vi "mymodule2.vi"() -> ()   [LabVIEW 2018]
uses:
  <vilib>/Enthought/Python Integration Toolkit/api/Unpack Double Array.vi
  <vilib>/Enthought/Python Integration Toolkit/Python Integration Toolkit.lvlib
panel:
  in  "停止":bool
  out "Data Out":dbl[](array[numeric])
  in  "OFFSET":dbl
  in  "Call Python":bool
  in  "Scale":dbl
  in  "Data In":dbl[](array[numeric])
  # "Python Global Varables"
  # "Data Out = Data In * Scale + OFFSET"
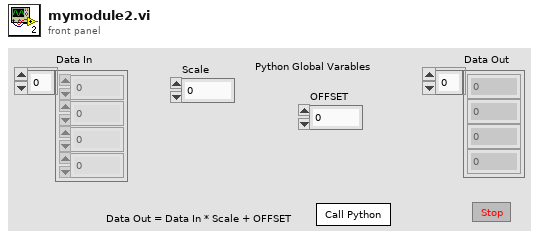
[diagram p1: front panel]
types:
  T1 = typedef "Python Integration Toolkit.lvlib/Session ID.ctl" = u64
  T2 = typedef "Python Integration Toolkit.lvlib/Python Objects.ctl" = variant
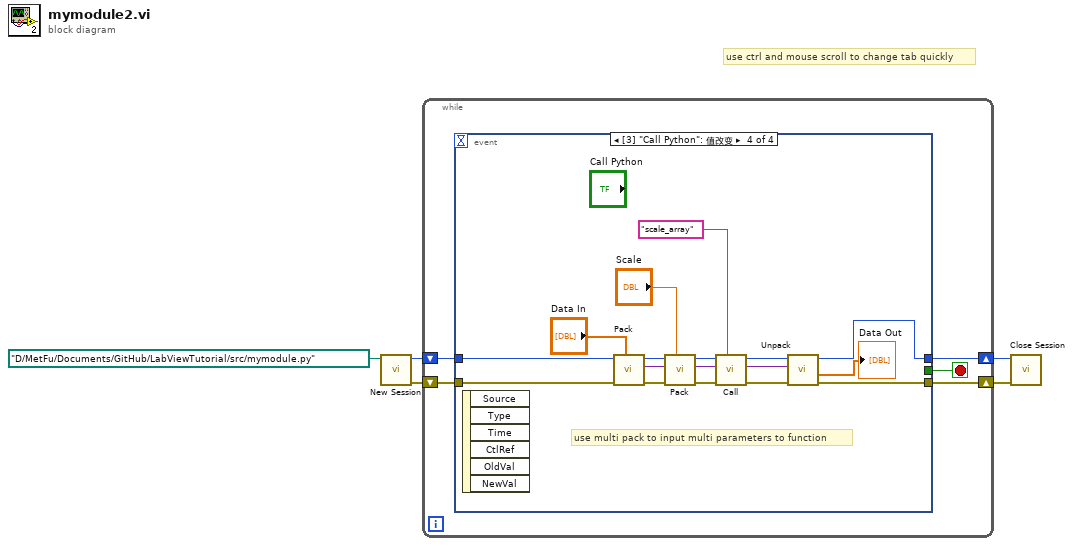
[diagram p0: block diagram]
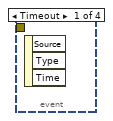
[diagram p2: hidden frame]
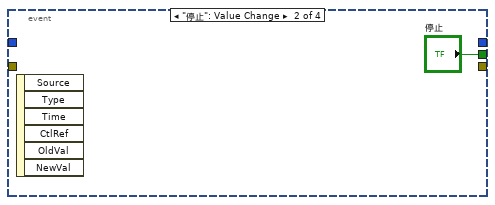
[diagram p3: hidden frame]
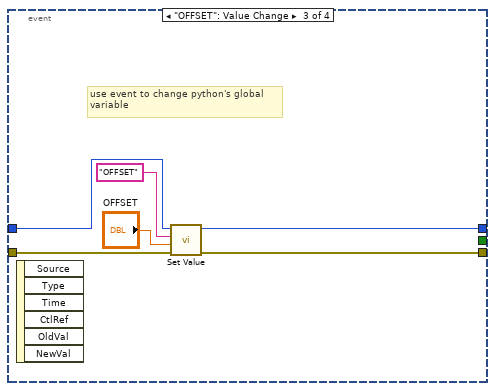
[diagram p4: hidden frame]
diagram:
  # "use ctrl and mouse scroll to change tab quickly"
  n1 = call <vilib>:"New Session.vi"("Path to Python Module (.py File)"=path "D:/MetFu/Documents/GitHub/LabViewTutorial/src/mymodule.py") -> ("error out"=w1:errorcluster, "Session ID out"=w4:T1)  [unwired: 9 in]
  n2 = while {
    shift-right: [w9] -> w3
    shift-left: w4 -> [w10]
    shift-right: [w8] -> w2
    shift-left: w1 -> [w7]
    stop <- w6 stop-if-true
    n3 = event shown="[3] \"Call Python\": 值改变" {
      selector: _ -> [_ _ _ _]
      dyn-events: _ -> [_ _ _ _]
      timeout: _ -> [_ _ _ _]
      tunnel: w10 -> [_ _ w15 w30]
      tunnel: [_ _ w14 w29] -> w9
      tunnel: [_ _ w13 w27] -> w8
      tunnel: w7 -> [_ _ w12 w28]
      tunnel: [_ "停止" _ _] -> w6
      event Timeout {
        n4 = event-data() -> ()  [unwired: 1 in, 3 out]
      }
      event "停止": Value Change {
        n5 = event-data() -> ()  [unwired: 1 in, 6 out]
      }
      event "OFFSET": Value Change {
        # "use event to change python's global\nvariable"
        n6 = event-data() -> ()  [unwired: 1 in, 6 out]
        n7 = call <vilib>:"Set Value.vi"("error in (no error)"=w12, "Value"="OFFSET", "Object Name"="OFFSET", "Session ID"=w15) -> ("error out"=w13:errorcluster, "Session ID out"=w14:T1)  [unwired: 6 in]
      }
      event "Call Python": Value Change {
        # "use multi pack to input multi parameters to function"
        n8 = event-data() -> ()  [unwired: 1 in, 6 out]
        n9 = call <vilib>:"Pack.vi"("Argument"="Data In", "error in (no error)"=w28, "Session ID"=w30) -> ("error out"=w20:errorcluster, "Python Object References Out"=w23:T2, "Session ID out"=w25:T1)  [unwired: 6 in]
        n10 = call <vilib>:"Pack.vi"("Argument"="Scale", "error in (no error)"=w20, "Python Object References In"=w23, "Session ID"=w25) -> ("error out"=w21:errorcluster, "Python Object References Out"=w22:T2, "Session ID out"=w24:T1)  [unwired: 5 in]
        n11 = call <vilib>:"Call.vi"("Function or Method Name"="scale_array", "error in (no error)"=w21, "Python Object References In"=w22, "Session ID"=w24) -> ("error out"=w33:errorcluster, "Python Object References Out"=w34:T2, "Session ID out"=w32:T1)  [unwired: 5 in]
        n12 = call-poly <vilib>:"Unpack.vi"("error in (no error)"=w33, "Python Object References In"=w34, "Session ID"=w32) -> ("error out"=w27:errorcluster, "Value"=→"Data Out":dbl[], "Session ID out"=w29:T1)  [unwired: 5 in, 1 out]
      }
    }
  }
  n13 = call <vilib>:"Close Session.vi"("error in (no error)"=w2, "Session ID"=w3) -> ()  [unwired: 9 in, 1 out]
